vi "写入VISA resource name.vi"(8 "error in (no error)":errorcluster caption="错误输入（无错误）", 10 "VISA resource name":refnum<visa-resource-name>, 11 "DP输入":refnum<class "DP.lvclass">) -> (0 "error out":errorcluster caption="错误输出", 3 "DP输出":refnum<class "DP.lvclass">)   [LabVIEW 2020, in "DP.lvlib" / "DP.lvclass"]
uses:
  DP.lvclass
  DP.lvclass/DP.ctl
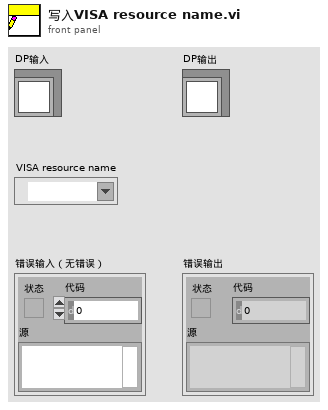
[diagram p1: front panel]
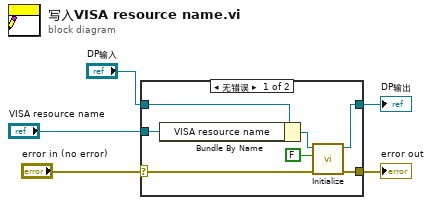
[diagram p0: block diagram]
diagram:
  n1 = case shown="无错误" "error in (no error)" {
    selector: "error in (no error)" -> [w12 w13]
    tunnel: [w9 w13] -> w4
    tunnel: [w7 w14] -> w2
    tunnel: "DP输入" -> [w11 w14]
    tunnel: "VISA resource name" -> [w10 _]
    frame No Error {
      n2 = Bundle By Name(cluster=w11, "VISA resource name"=w10) -> (w8:refnum<class "DP.lvclass">)
      n3 = call "Initialize.vi"("error in (no error)"=w12, "Reset? (T: Reset)"=FALSE, "DP 输入"=w8) -> ("error out"=w9:errorcluster, "DP 输出"=w7:refnum<class "DP.lvclass">)  [unwired: 7 in]
    }
    frame Error {
    }
  }
  "error out" <- w4
  "DP输出" <- w2
